vi "Match_Timer.vi"(8 "error in (no error)":errorcluster) -> ()   [LabVIEW 2018]
uses:
  <vilib>/Rock Robotics/Network Tables/NT Write String.vi
panel:
  out "Match Time":string
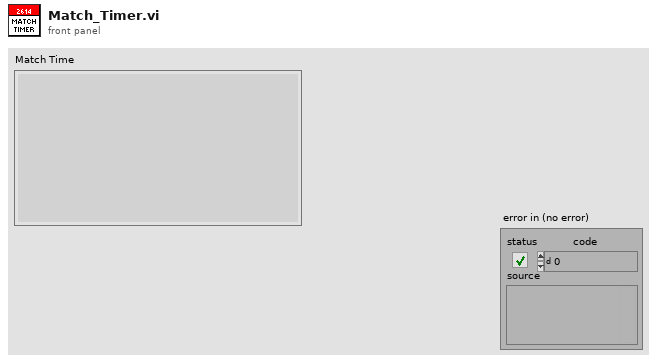
[diagram p1: front panel]
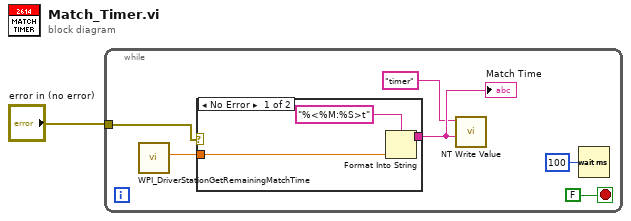
[diagram p0: block diagram]
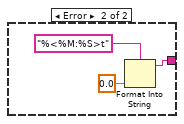
[diagram p2: hidden frame]
diagram:
  n1 = while {
    tunnel: "error in (no error)" -> [w2]
    stop <- FALSE stop-if-true
    n2 = call <vilib>:"WPI_DriverStationGetRemainingMatchTime.vi"() -> ("Match Time(s)"=w6:sgl)  [unwired: 10 in, 1 out]
    n3 = case shown="No Error" w2 {
      tunnel: w6 -> [w10 _]
      tunnel: [w8 w13] -> w7
      frame No Error {
        n4 = Format Into String(format string="%<%M:%S>t", w10) -> (resulting string=w8:string)  [unwired: 2 in, 1 out]
      }
      frame Error {
        n5 = Format Into String(format string="%<%M:%S>t", sgl 0.0 ("input 1")) -> (resulting string=w13:string)  [unwired: 2 in, 1 out]
      }
    }
    "Match Time" <- w7
    n6 = call-poly <vilib>:"NT Write Value.vi"("String"=w7, "Name"="timer") -> ()  [unwired: 9 in, 1 out]
    n7 = Wait (ms)(milliseconds to wait=u32 100) -> ()  [unwired: 1 out]
  }
